vi "Get Result.vi"(6 "Last request":bool, 8 "error in (no error)":errorcluster, 11 "Instrument Recorder in":refnum<class "Instrument Actor.lvclass">) -> (0 "error out":errorcluster, 2 "Result":refnum<class "Acquired Result.lvclass">, 3 "Instrument Recorder out":refnum<class "Instrument Actor.lvclass">)   [LabVIEW 2016, in "Instrument Actor.lvclass"]
uses:
  Instrument Actor.lvclass
  C:/github/LabActor/Worker/Worker.lvclass
  NHMFL_Core/Libraries/Instruments/Results/Acquired Result/Acquired Result.lvclass
  Instrument Actor.lvclass/Instrument Actor.ctl
  Worker/Worker.lvclass/Worker.ctl
  NHMFL_Core/Libraries/Instruments/Instrument Driver/Instrument Driver.lvclass/Instrument Driver.ctl
  Read Instrument driver.vi
  Worker/Read Cycle count.vi
  NHMFL_Core/Libraries/Instruments/Instrument Driver/Write Cycle count.vi
  Write Instrument driver.vi
  NHMFL_Core/Libraries/Instruments/Instrument Driver/Instrument Driver.lvclass
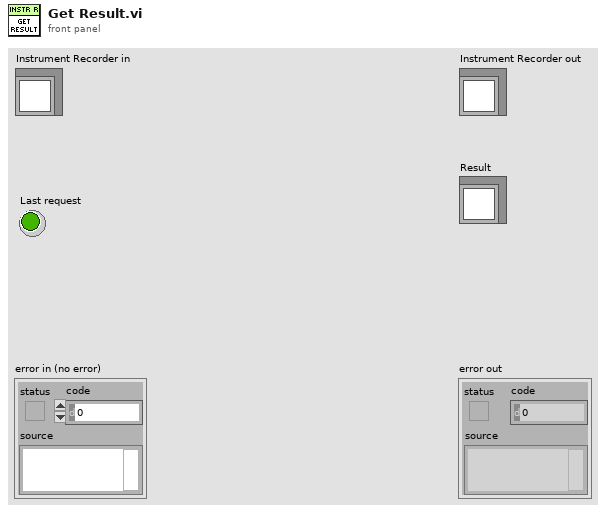
[diagram p1: front panel]
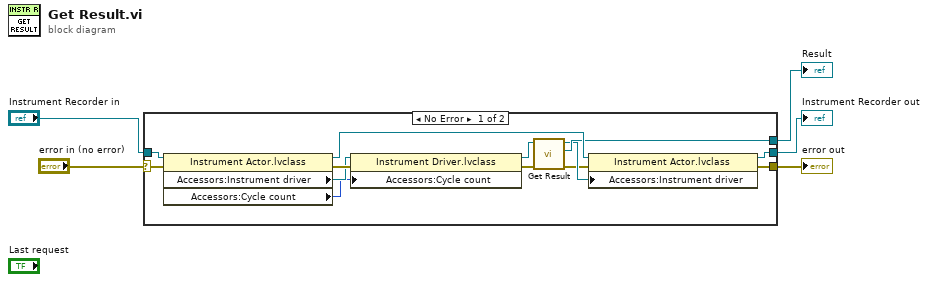
[diagram p0: block diagram]
diagram:
  n1 = case shown="No Error" "error in (no error)" {
    selector: "error in (no error)" -> [w12 w20]
    tunnel: [w10 w20] -> w4
    tunnel: [w15 w19] -> w2
    tunnel: "Instrument Recorder in" -> [w18 w19]
    tunnel: [w16 _] -> w1
    frame No Error {
      n2 = property class="Instrument Actor.lvclass"(reference=w18, error in=w12) -> (reference out=w17:refnum<class "Instrument Actor.lvclass">, error out=w13:errorcluster, "Accessors:Instrument driver"=w8:refnum<class "Instrument Driver.lvclass">, "Accessors:Cycle count"=w6:i32)
      n3 = property class="Instrument Driver.lvclass"(reference=w8, error in=w13, "Accessors:Cycle count"=w6) -> (reference out=w7:refnum<class "Instrument Driver.lvclass">, error out=w9:errorcluster)
      n4 = call-dynamic "Get Result.vi"("error in (no error)"=w9, "Instrument Driver in"=w7) -> ("error out"=w11:errorcluster, "Result"=w16:refnum<class "Acquired Result.lvclass">, "Instrument Driver out"=w14:refnum<class "Instrument Driver.lvclass">)  [unwired: 7 in]
      n5 = property class="Instrument Actor.lvclass"(reference=w17, error in=w11, "Accessors:Instrument driver"=w14) -> (reference out=w15:refnum<class "Instrument Actor.lvclass">, error out=w10:errorcluster)
    }
    frame Error {
    }
  }
  "error out" <- w4
  "Instrument Recorder out" <- w2
  "Result" <- w1
